vi "SUB-확인 메세지.vi"(2 "타임아웃(ms)":i32, 3 "메세지":string) -> ()   [LabVIEW 2015]
panel:
  out "카운터":u32=1000
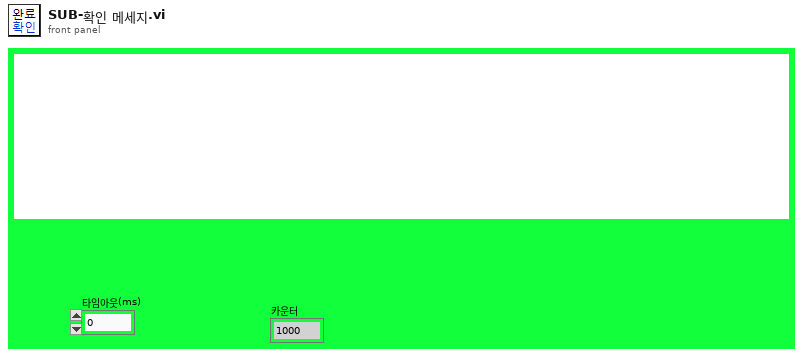
[diagram p1: front panel]
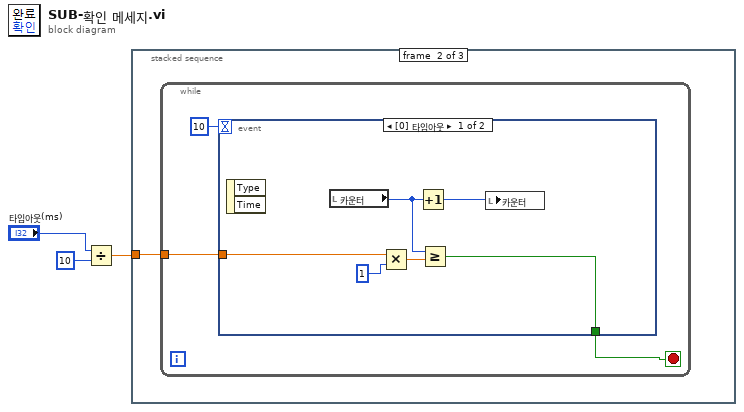
[diagram p0: block diagram]
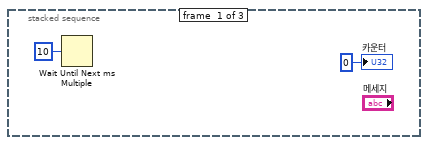
[diagram p2: hidden frame]
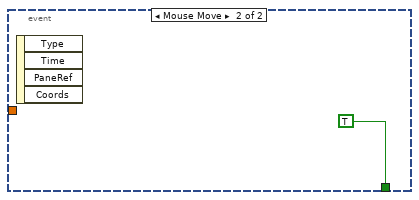
[diagram p3: hidden frame]
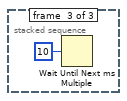
[diagram p4: hidden frame]
diagram:
  n1 = Divide(x="타임아웃(ms)", y=10) -> (x/y=w1:dbl)
  n2 = stacked-sequence {
    tunnel: w1 -> [_ w6 _]
    frame #0 {
      n3 = Wait Until Next ms Multiple(millisecond multiple=u32 10 ("ms 배수")) -> ()  [unwired: 1 out]
      "카운터" <- u32 0 ("카운터")
    }
    frame #1 {
      n4 = while {
        tunnel: w6 -> [w7]
        stop <- w9 stop-if-true
        n5 = event shown="[0] 타임아웃" {
          selector: _ -> [_ _]
          dyn-events: _ -> [_ _]
          timeout: 10 -> [_ _]
          tunnel: [w11 TRUE] -> w9
          tunnel: w7 -> [w10 _]
          event Timeout {
            n6 = event-data() -> ()  [unwired: 1 in, 2 out]
            n7 = local read "카운터"() -> (w14:u32)
            n8 = Multiply(x=w10, y=1) -> (x*y=w13:dbl)
            n9 = Increment(x=w14) -> (x+1=w15:u32)
            n10 = Greater Or Equal?(x=w14, y=w13) -> (x >= y?=w11:bool)
            n11 = local write "카운터"(w15) -> ()
          }
          event Mouse Move {
            n12 = event-data() -> ()  [unwired: 1 in, 4 out]
          }
        }
      }
    }
    frame #2 {
      n13 = Wait Until Next ms Multiple(millisecond multiple=u32 10 ("ms 배수")) -> ()  [unwired: 1 out]
    }
  }
